vi "postPubDataSV.vi"(6 "newValue (T)":bool=TRUE, 8 "error in (no error)":errorcluster, 9 "value":variant, 10 "pubDataSV":T1=enum."LoopTime_ms", 11 "MiddlewareSVThisComponent in":refnum<class "MiddlewareSVThisComponent.lvclass">) -> (0 "error out":errorcluster, 3 "MiddlewareSVThisComponent out":refnum<class "MiddlewareSVThisComponent.lvclass">)   [LabVIEW 2015, in "MiddlewareSVThisComponent.lvclass"]
uses:
  MiddlewareSVThisComponent.lvclass
  Typedefs/PubDataSV.ctl
  Typedefs/EXATypedefs.lvlib
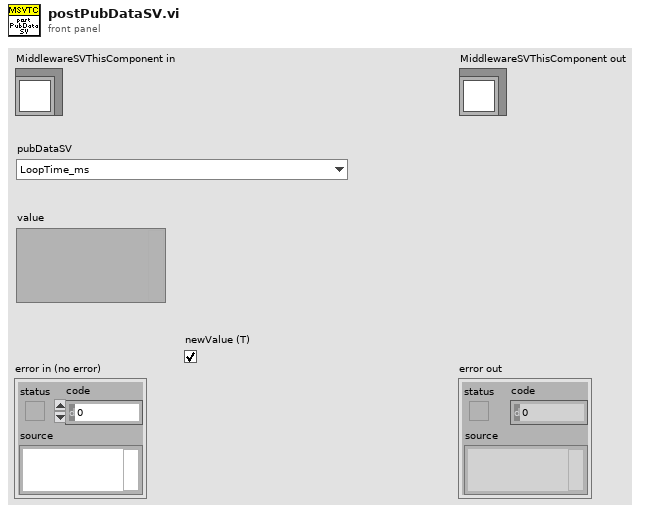
[diagram p1: front panel]
types:
  T1 = typedef "EXATypedefs.lvlib/PubDataSV.ctl" = enum16{"DetailedState", "ErrorCode", "Heartbeat", "LoopTime_ms", "LoopTimeOutOfRange", "RejectedCommand", "SummaryState", "Timestamp"}
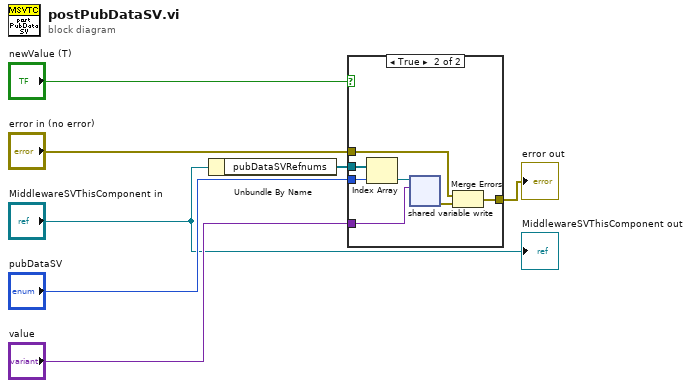
[diagram p0: block diagram]
diagram:
  n1 = Unbundle By Name("MiddlewareSVThisComponent in") -> ("pubDataSVRefnums"=w6:refnum<k21>[])
  n2 = case shown="True" "newValue (T)" {
    tunnel: w6 -> [_ w15]
    tunnel: "pubDataSV" -> [_ w14]
    tunnel: "value" -> [_ w11]
    tunnel: "error in (no error)" -> [w8 w10]
    tunnel: [w8 w12] -> w1
    frame False {
    }
    frame True {
      n3 = Index Array(array=w15, index=w14) -> (element=w13:refnum<k21>)
      n4 = shared-variable-write(w13, w11) -> (w9:errorcluster)  [unwired: 1 in, 1 out]
      n5 = Merge Errors(w10, w9) -> (w12:errorcluster)
    }
  }
  "error out" <- w1
  "MiddlewareSVThisComponent out" <- "MiddlewareSVThisComponent in"
